vi "FetchTargetFolder.vi"(7 "Use default Folder":bool, 11 "Target Folder":path) -> (0 "error out":errorcluster, 3 "Full File Path":path)   [LabVIEW 2018, in "RW_Protocols.lvlib"]
uses:
  RW_Protocols.lvlib
panel:
  out "file or folder exists?":bool
  out "Is Path and Not Empty?":bool
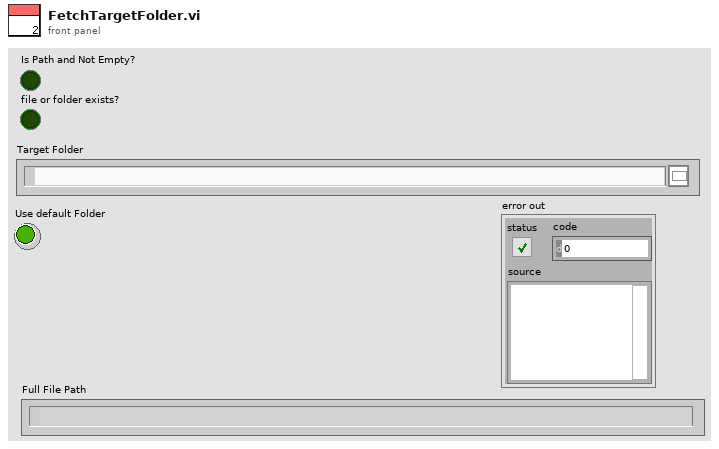
[diagram p1: front panel]
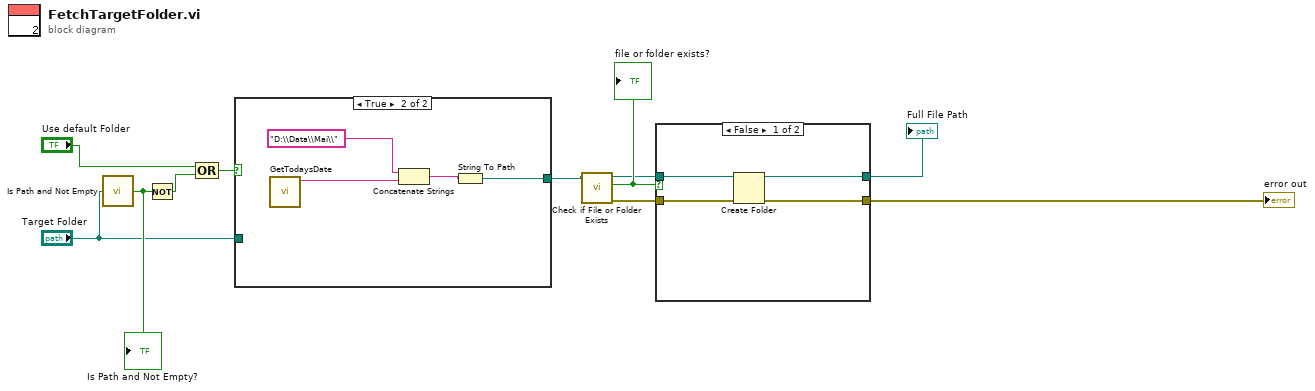
[diagram p0: block diagram]
diagram:
  n1 = call <vilib>:"Is Path and Not Empty.vi"("path"="Target Folder") -> ("Is Path and Not Empty?"=w4:bool)  [unwired: 4 in]
  "Is Path and Not Empty?" <- w4
  n2 = Not(x=w4) -> (.not. x?=w5:bool)
  n3 = Compound Arithmetic op=OR("Use default Folder", w5) -> (w1:bool)
  n4 = case shown="True" w1 {
    tunnel: [w12 w13] -> w11
    tunnel: "Target Folder" -> [w12 _]
    frame False {
    }
    frame True {
      n5 = call "GetTodaysDate.vi"() -> ("concatenated string"=w15:string)  [unwired: 10 in, 1 out]
      n6 = Concatenate Strings("D:\\Data\\Mai\\", w15) -> (w14:string)
      n7 = String To Path(string=w14) -> (path=w13:path)
    }
  }
  n8 = call <vilib>:"Check if File or Folder Exists.vi"("path"=w11) -> ("error out"=w7:errorcluster, "file or folder exists?"=w10:bool, "dup path"=w9:path)  [unwired: 8 in]
  "file or folder exists?" <- w10
  n9 = case shown="False" w10 {
    tunnel: w9 -> [w20 w22]
    tunnel: [w19 w22] -> w8
    tunnel: w7 -> [w18 w21]
    tunnel: [w17 w21] -> w2
    frame False {
      n10 = Create Folder(path (use dialog)=w20, error in=w18) -> (created path=w19:path, error out=w17:errorcluster)  [unwired: 1 in, 1 out]
    }
    frame True {
    }
  }
  "Full File Path" <- w8
  "error out" <- w2
